vi "Limit Position Read.vi"(4 "error in (no error)":errorcluster, 6 "Container State":T2, 7 "Display State In":T1={"Numeric"=0.0, "Fill Plots"=FALSE, "Cursor Redraw"=TRUE, "XYGraph Refnum"=refnum}) -> (0 "error out":errorcluster, 2 "Value":cluster{"Lower Limit":dbl, "Upper Limit":dbl}, 3 "Display State Out":T1={"Numeric"=0.0, "Fill Plots"=FALSE, "Cursor Redraw"=TRUE, "XYGraph Refnum"=refnum})   [LabVIEW 2020, in "Overview XControl.xctl"]
uses:
  Overview XControl.xctl
  <vilib>/_xctls/Container State.ctl
  Overview State.ctl
  <vilib>/_xctls/XControlSupport.lvlib
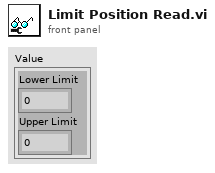
[diagram p1: front panel]
types:
  T1 = typedef "Overview XControl.xctl/Overview State.ctl" = cluster{"Numeric":dbl, "Fill Plots":bool, "Cursor Redraw":bool, "XYGraph Refnum":refnum<vi>}
  T2 = typedef "XControlSupport.lvlib/Container State.ctl" = cluster{"Indicator?":bool, "Run Mode?":bool, " Refnum":refnum<vi>}
  T3 = cluster{"Cursor.Cursor X":dbl, "Cursor.Cursor X":dbl}
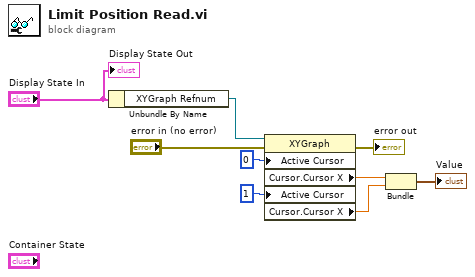
[diagram p0: block diagram]
diagram:
  n1 = Unbundle By Name("Display State In") -> ("XYGraph Refnum"=w6:refnum<vi>)
  n2 = property class="XYGraph"(reference=w6, error in="error in (no error)", "Active Cursor"=u32 0, "Active Cursor"=u32 1) -> (error out=→"error out":errorcluster, "Cursor.Cursor X"=w5:dbl, "Cursor.Cursor X"=w4:dbl)  [unwired: 1 out]
  n3 = Bundle("Cursor.Cursor X"=w5, "Cursor.Cursor X"=w4) -> (→"Value":T3)  [unwired: 1 in]
  "Display State Out" <- "Display State In"
